vi "Calculate Multipoint Calibration(RT).vi"(0 "X":dbl[](array[numeric]), 7 "Y":dbl[](array[numeric]), 11 "Tolerance":dbl=1.0 format="%#_13g") -> (4 "Results":dbl[](array[numeric]), 8 "Poly. Coefficients":dbl[](array[numeric]), 15 "Valid?":bool)   [LabVIEW 2013]
uses:
  <vilib>/Analysis/NI_AALPro.lvlib
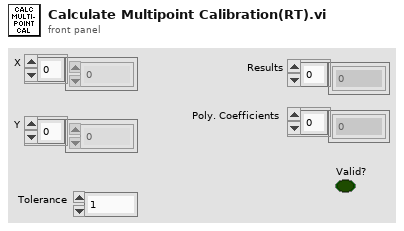
[diagram p1: front panel]
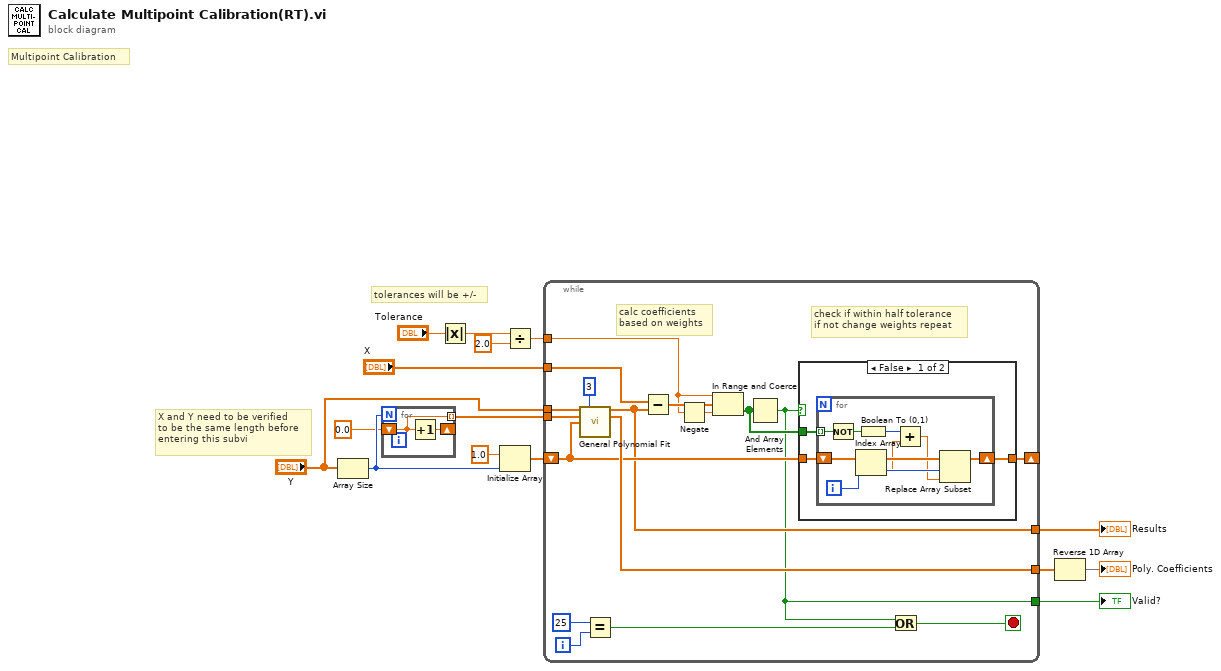
[diagram p0: block diagram]
diagram:
  # "tolerances will be +/-"
  # "X and Y need to be verified\nto be the same length before\nentering this subvi"
  # "Multipoint Calibration"
  n1 = Array Size(array="Y") -> (size(s)=w6:i32)
  n2 = for {
    N: w6 -> [_]
    shift-right: [w17] -> _
    shift-left: 0.0 ("element") -> [w16]
    tunnel: [w16] -> w4 mode=indexing
    n3 = Increment(x=w16) -> (x+1=w17:dbl)
  }
  n4 = Absolute Value(x="Tolerance") -> (abs(x)=w12:dbl)
  n5 = Initialize Array(1.0 ("element"), w6) -> (w14:dbl[])
  n6 = Divide(x=w12, y=2.0) -> (x/y=w10:dbl)
  n7 = while {
    tunnel: "Y" -> [w33]
    shift-right: [w27] -> _
    shift-left: w14 -> [w28]
    tunnel: [w32] -> w2
    tunnel: w10 -> [w29]
    tunnel: [w25] -> w9
    tunnel: [w20] -> w8
    tunnel: "X" -> [w19]
    tunnel: w4 -> [w18]
    i -> [w23]
    stop <- w21 stop-if-true
    # "check if within half tolerance\nif not change weights repeat"
    # "calc coefficients\nbased on weights"
    n8 = call <vilib>:"General Polynomial Fit.vi"("Y"=w33, "polynomial order"=3, "X"=w18, "Weight"=w28) -> ("Best Polynomial Fit"=w25:dbl[], "Polynomial Coefficients"=w32:dbl[])  [unwired: 8 in, 2 out]
    n9 = Equal?(x=25 ("polynomial order"), y=w23) -> (x = y?=w22:bool)
    n10 = Subtract(x=w19, y=w25) -> (x-y=w31:dbl[])
    n11 = Negate(x=w29) -> (-x=w30:dbl)
    n12 = In Range and Coerce(upper limit=w29, x=w31, lower limit=w30) -> (In Range?=w26:bool[])  [unwired: 1 out]
    n13 = And Array Elements(Boolean array=w26) -> (logical AND=w20:bool)
    n14 = case shown="False" w20 {
      tunnel: [w35 w46] -> w27
      tunnel: w28 -> [w37 w46]
      tunnel: w26 -> [w36 _]
      frame False {
        n15 = for {
          tunnel: w36 -> [w41] mode=indexing
          shift-right: [w38] -> w35
          shift-left: w37 -> [w45]
          i -> [w44]
          n16 = Not(x=w41) -> (.not. x?=w40:bool)
          n17 = Index Array(array=w45, index=w44) -> (element=w43:dbl)
          n18 = Boolean To (0,1)(Boolean=w40) -> (0, 1=w42:i16)
          n19 = Add(x=w42, y=w43) -> (x+y=w39:dbl)
          n20 = Replace Array Subset(array=w45, new element=w39, index=w44) -> (w38:dbl[])
        }
      }
      frame True {
      }
    }
    n21 = Or(x=w20, y=w22) -> (x .or. y?=w21:bool)
  }
  "Results" <- w9
  "Valid?" <- w8
  n22 = Reverse 1D Array(array=w2) -> (reversed array=→"Poly. Coefficients":dbl[])
